vi "Pneumatic Main.vi"(11 "Control Mode":enum16{"Open", "Control"}(ring)) -> ()   [LabVIEW 2018]
uses:
  <vilib>/Rock Robotics/WPI/Solenoid/WPI_SolenoidChannel.ctl
  <vilib>/Rock Robotics/WPI/Solenoid/WPI_SolenoidDevRef.ctl
  <vilib>/Rock Robotics/WPI/Compressor/WPI_CompressorDevRef.ctl
  <vilib>/Rock Robotics/WPI/Solenoid/WPI_SolenoidValue.ctl
  <vilib>/Rock Robotics/WPI/Solenoid/WPI_SolenoidOpenSingle.vi
  <vilib>/Rock Robotics/WPI/Utilities/WPI_GetSetVariantRefNum.vi
  Robot Global Data.vi
  <vilib>/Rock Robotics/WPI/Solenoid/WPI_SolenoidSetEnum.vi
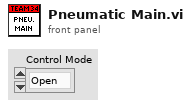
[diagram p1: front panel]
types:
  T1 = typedef "WPI_SolenoidDevRef.ctl" = cluster{"DevStatus":errorcluster, "Pneumatics Control Module":u8, "Forward Solenoid Channel":T2, "Reverse Solenoid Channel":T2}
  T2 = typedef "WPI_SolenoidChannel.ctl" = enum8{"Solenoid 0", "Solenoid 1", "Solenoid 2", "Solenoid 3", "Solenoid 4", "Solenoid 5", "Solenoid 6", "Solenoid 7", "Invalid"}
  T3 = typedef "WPI_CompressorDevRef.ctl" = cluster{"DevStatus":errorcluster, "Pneumatics Control Module":u8}
  T4 = typedef "WPI_SolenoidValue.ctl" = enum16{"Off", "On", "Forward", "Reverse"}
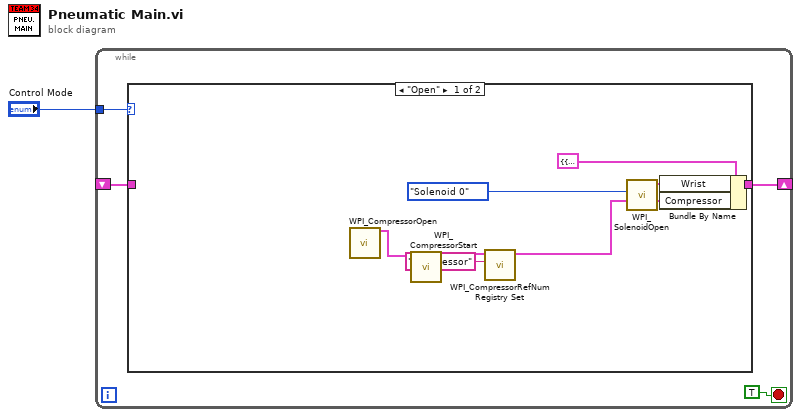
[diagram p0: block diagram]
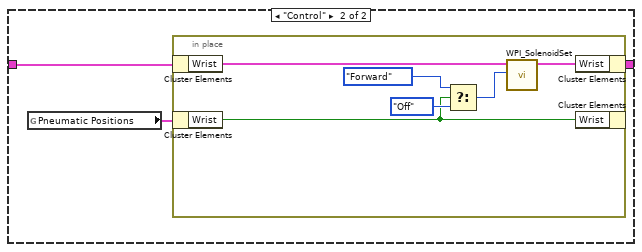
[diagram p2: hidden frame]
diagram:
  n1 = while {
    tunnel: "Control Mode" -> [w4]
    shift-right: [w2] -> _
    shift-left: _ -> [w3]
    stop <- TRUE stop-if-true
    n2 = case shown="\"Open\"" w4 {
      tunnel: w3 -> [_ w15]
      tunnel: [w11 w14] -> w2
      frame "Open" {
        n3 = call <vilib>:"WPI_CompressorOpen.vi"() -> ("CompressorDevRef"=w9:T3)  [unwired: 14 in, 1 out]
        n4 = call <vilib>:"WPI_CompressorStart.vi"("CompressorDevRef"=w9) -> ("CompressorDevRef"=w8:T3)  [unwired: 9 in, 1 out]
        n5 = call <vilib>:"WPI_CompressorRefNum Registry Set.vi"("refnum name"="compressor", "CompressorDevRef"=w8) -> ("CompressorDevRef"=w7:T3)  [unwired: 8 in, 1 out]
        n6 = call-poly <vilib>:"WPI_SolenoidOpen.vi"("Solenoid Channel"=WPI_SolenoidChannel."Solenoid 0") -> ("SolenoidDevRef"=w10:T1)  [unwired: 9 in, 1 out]
        n7 = Bundle By Name(cluster=cluster{"Wrist":T1, "Compressor":T3} {"Wrist"={"DevStatus"={"status"=FALSE, "code"=0, "source"=""}, "Pneumatics Control Module"=0, "Forward Solenoid Channel"=enum."Invalid", "Reverse Solenoid Channel"=enum."Invalid"}, "Compressor"={"DevStatus"={"status"=FALSE, "code"=0, "source"=""}, "Pneumatics Control Module"=0}} ("input cluster"), "Wrist"=w10, "Compressor"=w7) -> (w11:cluster{"Wrist":T1, "Compressor":T3})
      }
      frame "Control" {
        n8 = global read "Robot Global Data.vi" "Pneumatic Positions"() -> (w16:cluster{"Wrist":bool})
        n9 = in-place {
          n10 = in-place-cluster #1(w15) -> ("Wrist"=w19:T1)
          n11 = in-place-cluster #2(w16) -> ("Wrist"=w17:bool)
          n12 = Select(t=WPI_SolenoidValue."Forward" ("Value"), s=w17, f=WPI_SolenoidValue."Off") -> (s? t:f=w20:T4)
          n13 = call-poly <vilib>:"WPI_SolenoidSet.vi"("Value"=w20, "SolenoidDevRef"=w19) -> ("SolenoidDevRef"=w18:T1)  [unwired: 8 in, 1 out]
          n14 = in-place-cluster #1("Wrist"=w18) -> (w14:cluster{"Wrist":T1, "Compressor":T3})
          n15 = in-place-cluster #2("Wrist"=w17) -> ()  [unwired: 1 out]
        }
      }
    }
  }
